vi "Half_FULL_ADDER.vi"() -> ()   [LabVIEW 2026]
panel:
  in  "C_in":bool
  out "COUT":bool
  out "SUM":bool
  in  "B":bool
  in  "A":bool
  out "CARRY":bool
  out "SUM":bool
  in  "i/p B":bool
  in  "i/p A":bool
  # "HALD-ADDER"
  # "FULL-ADDER"
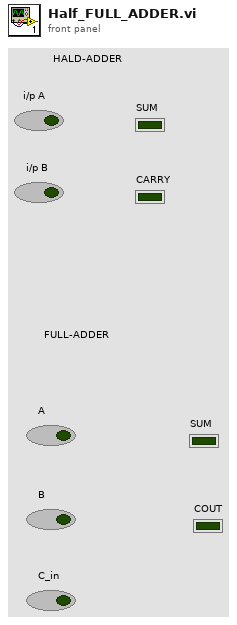
[diagram p1: front panel]
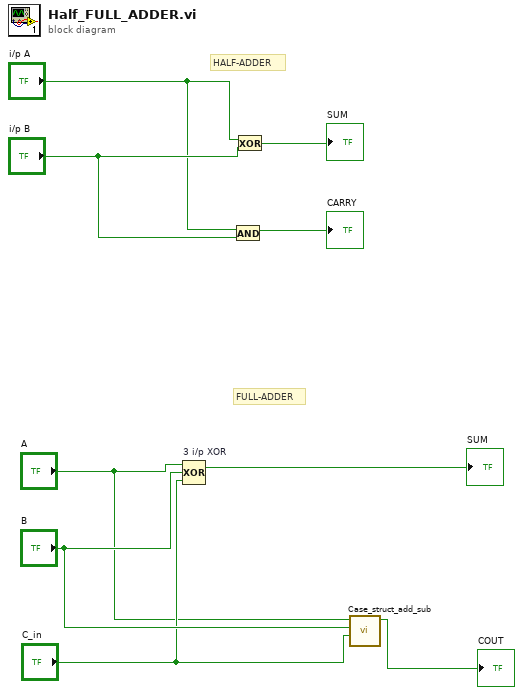
[diagram p0: block diagram]
diagram:
  # "FULL-ADDER"
  # "HALF-ADDER"
  n1 = Compound Arithmetic op=XOR "3 i/p XOR"("A", "B", "C_in") -> (→"SUM":bool)
  n2 = And(x="i/p A", y="i/p B") -> (x .and. y?=→"CARRY":bool)
  n3 = Exclusive Or(1:"i/p B", 2:"i/p A") -> (0:→"SUM":bool)
  n4 = call "Case_struct_add_sub.vi"("C_in"="C_in", "B"="B", "A"="A") -> ("Boolean"=→"COUT":bool)  [unwired: 8 in]
